vi "20211008_Event structure.vi"() -> ()   [LabVIEW 2019]
panel:
  out "current time":timestamp
  in  "millisecond multiple":u32(knob) scale=1.0..10000.0
  out "Numeric 2":i32
  in  "stop":bool
  out "Numeric":dbl
  in  "Knob":u32(knob) scale=0.0..9.0
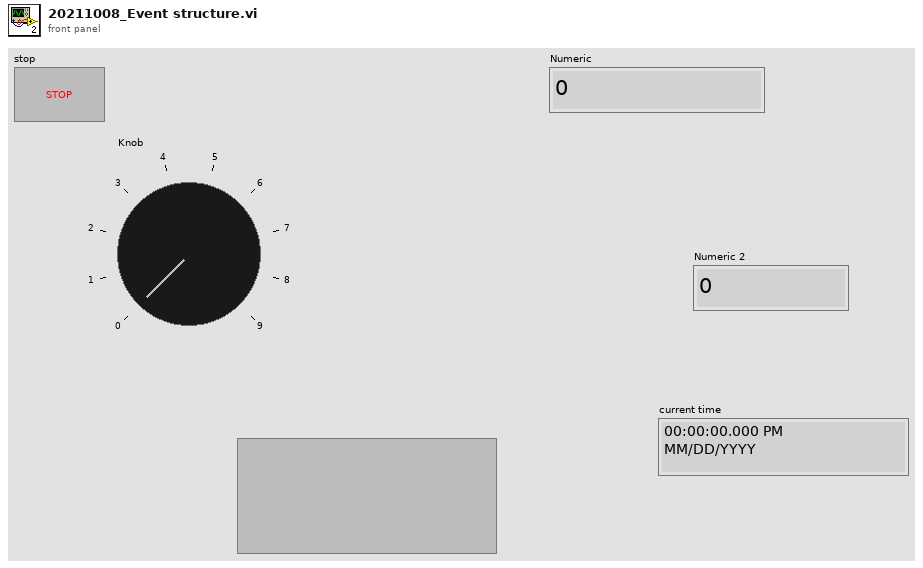
[diagram p1: front panel]
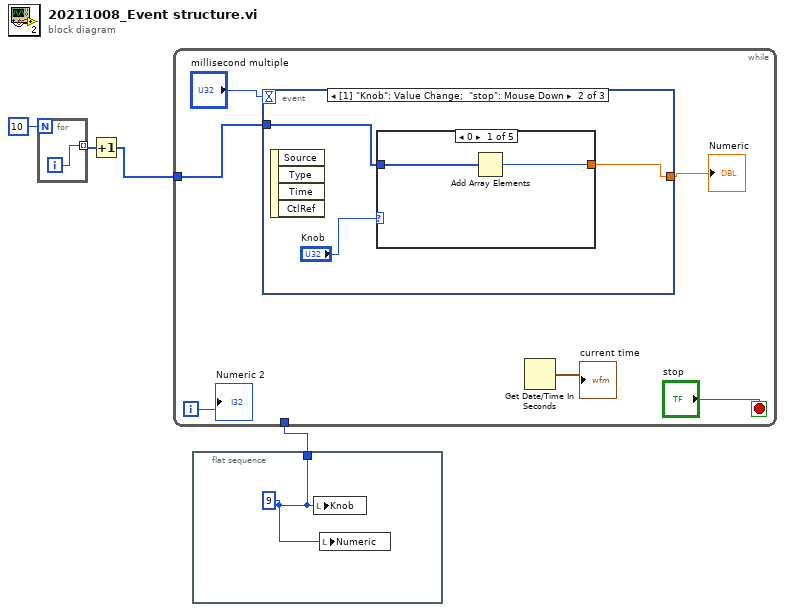
[diagram p0: block diagram]
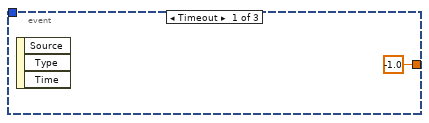
[diagram p2: hidden frame]
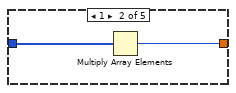
[diagram p3: hidden frame]
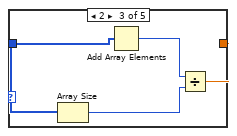
[diagram p4: hidden frame]
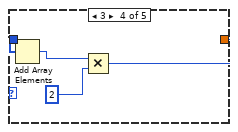
[diagram p5: hidden frame]
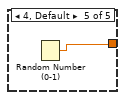
[diagram p6: hidden frame]
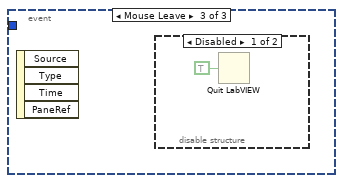
[diagram p7: hidden frame]
diagram:
  n1 = for {
    N: 10 -> [_]
    tunnel: [w5] -> w3 mode=indexing
    i -> [w5]
  }
  n2 = Increment(x=w3) -> (x+1=w2:i32[])
  n3 = while {
    tunnel: w2 -> [w9]
    tunnel: w1 -> [_]
    i -> [w7]
    stop <- "stop" stop-if-true
    n4 = event shown="[1] \"Knob\": Value Change;  \"stop\": Mouse Down" {
      selector: _ -> [_ _ _]
      dyn-events: _ -> [_ _ _]
      timeout: "millisecond multiple" -> [_ _ _]
      tunnel: [-1.0 ("number: 0 to 1") w15 _] -> w10
      tunnel: w9 -> [_ w14 _]
      event Timeout {
        n5 = event-data() -> ()  [unwired: 1 in, 3 out]
      }
      event "Knob": Value Change; "stop": Mouse Down {
        n6 = event-data() -> ()  [unwired: 1 in, 4 out]
        n7 = case shown="0" "Knob" {
          tunnel: w14 -> [w17 w19 w23 w27 _]
          tunnel: [w16 w18 w20 w24 w28] -> w15
          frame 0 {
            n8 = Add Array Elements(numeric array=w17) -> (sum=w16:i32)
          }
          frame 1 {
            n9 = Multiply Array Elements(1:w19) -> (0:w18:i32)
          }
          frame 2 {
            n10 = Array Size(array=w23) -> (size(s)=w22:i32)
            n11 = Add Array Elements(numeric array=w23) -> (sum=w21:i32)
            n12 = Divide(x=w21, y=w22) -> (x/y=w20:dbl)
          }
          frame 3 {
            n13 = Add Array Elements(numeric array=w27) -> (sum=w26:i32)
            n14 = Multiply(x=w26, y=2) -> (x*y=w24:i32)
          }
          frame 4, Default {
            n15 = Random Number (0-1)() -> (number: 0 to 1=w28:dbl)
          }
        }
      }
      event Mouse Leave {
        n16 = event-data() -> ()  [unwired: 1 in, 4 out]
        n17 = disable-structure shown="Disabled" {
          frame Disabled {
            n18 = Quit LabVIEW(quit? (T)=TRUE ("stop? (T)")) -> ()
          }
          frame Enabled {
          }
        }
      }
    }
    "Numeric" <- w10
    n19 = Get Date/Time In Seconds() -> (seconds since 1Jan1904=→"current time":timestamp)
    "Numeric 2" <- w7
  }
  n20 = flat-sequence {
    tunnel: [w30] -> w1
    frame #0 {
      w30 = u32 9 ("Knob")
      n21 = local write "Knob"(w30) -> ()
      n22 = local write "Numeric"(w30) -> ()
    }
  }
